vi "例4-26.vi"() -> ()   [LabVIEW 2019]
panel:
  out "波形图":cluster{"X0":i32, "DeltaX":i32, dbl[]}(graph)
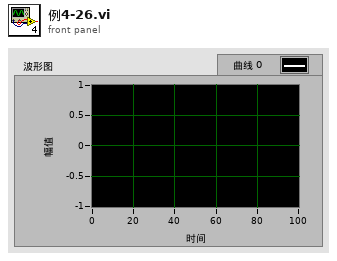
[diagram p1: front panel]
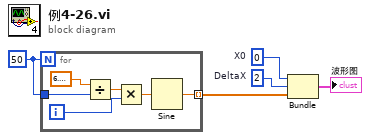
[diagram p0: block diagram]
diagram:
  w3 = 2  # DeltaX
  w4 = 0  # X0
  w5 = 50
  n1 = for {
    N: w5 -> [_]
    tunnel: w5 -> [w8]
    tunnel: [w6] -> w2 mode=indexing
    i -> [w7]
    n2 = Divide(x=6.283185307179586, y=w8) -> (x/y=w10:dbl)
    n3 = Multiply(x=w10, y=w7) -> (x*y=w9:dbl)
    n4 = Sine(x=w9) -> (sin(x)=w6:dbl)
  }
  n5 = Bundle("X0"=w4, "DeltaX"=w3, w2) -> (→"波形图":cluster{"X0":i32, "DeltaX":i32, dbl[]})  [unwired: 1 in]
